vi "ABR-Initialize Stimulus.vi"(0 "Data folder":path, 5 "Npts":i32, 7 "Stimulus":T1={"Destination"="", "Waveform"=enum."TONE PIP", "Frequency (kHz)"=16.0, "Rep rate (/sec)"=30.0, "Alternate Polarity"=FALSE, "Sampling rate (Hz)"=100000.0, "Duration (ms)"=5.0, "Ramp (ms)"=0.5, "Click width (us)"=0.0, "ITI"=enum."Rate"} {"Frequency (kHz)" format="%.2f"}, 11 "error in (no error)":errorcluster) -> (4 "SigMan out":refnum<class "SignalManager.lvclass">, 15 "error out":errorcluster)   [LabVIEW 2020]
uses:
  epl-vi-lib/Signal Synthesis VIs/4th Generation/Classes/SignalManager/SignalManager.lvclass
  Typedefs/ABR-Stimulus.ctl
  epl-vi-lib/Signal Synthesis VIs/4th Generation/Classes/Channel/Channel.lvclass/Channel.ctl
  epl-vi-lib/Signal Synthesis VIs/4th Generation/Classes/Channel/Write Waveform.vi
  epl-vi-lib/Signal Synthesis VIs/4th Generation/Classes/Channel/Write Gate.vi
  epl-vi-lib/Signal Synthesis VIs/4th Generation/Classes/Channel/Write Level.vi
  epl-vi-lib/Signal Synthesis VIs/4th Generation/Classes/Channel/Write AltPol.vi
  epl-vi-lib/Signal Synthesis VIs/4th Generation/Classes/Waveforms/Tone/Tone.lvclass
  D:/Development/epl-vi-lib/Signal Synthesis VIs/4th Generation/Classes/Waveforms/Waveform/Waveform.lvclass
  epl-vi-lib/Signal Synthesis VIs/4th Generation/Classes/Waveforms/Pulse Train/Pulse Train.lvclass
  epl-vi-lib/Signal Synthesis VIs/4th Generation/Classes/Channel/Channel.lvclass
  epl-vi-lib/Signal Synthesis VIs/4th Generation/Classes/Level/Level.lvclass
  epl-vi-lib/Signal Synthesis VIs/4th Generation/Classes/Gate/Gate.lvclass
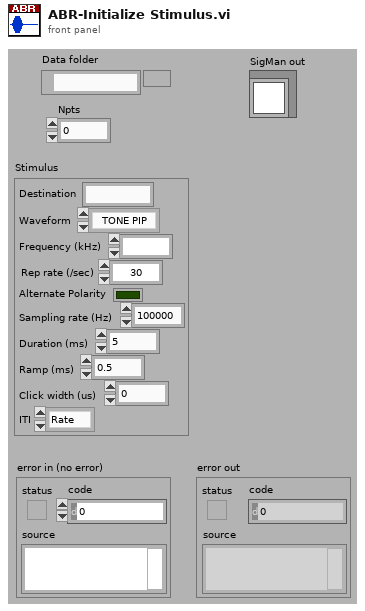
[diagram p1: front panel]
types:
  T1 = typedef "ABR-Stimulus.ctl" = cluster{"Destination":string, "Waveform":enum16{"TONE PIP", "CLICK"}, "Frequency (kHz)":ext, "Rep rate (/sec)":dbl, "Alternate Polarity":bool, "Sampling rate (Hz)":dbl, "Duration (ms)":dbl, "Ramp (ms)":dbl, "Click width (us)":dbl, "ITI":enum16{"Rate", "Interval"}}
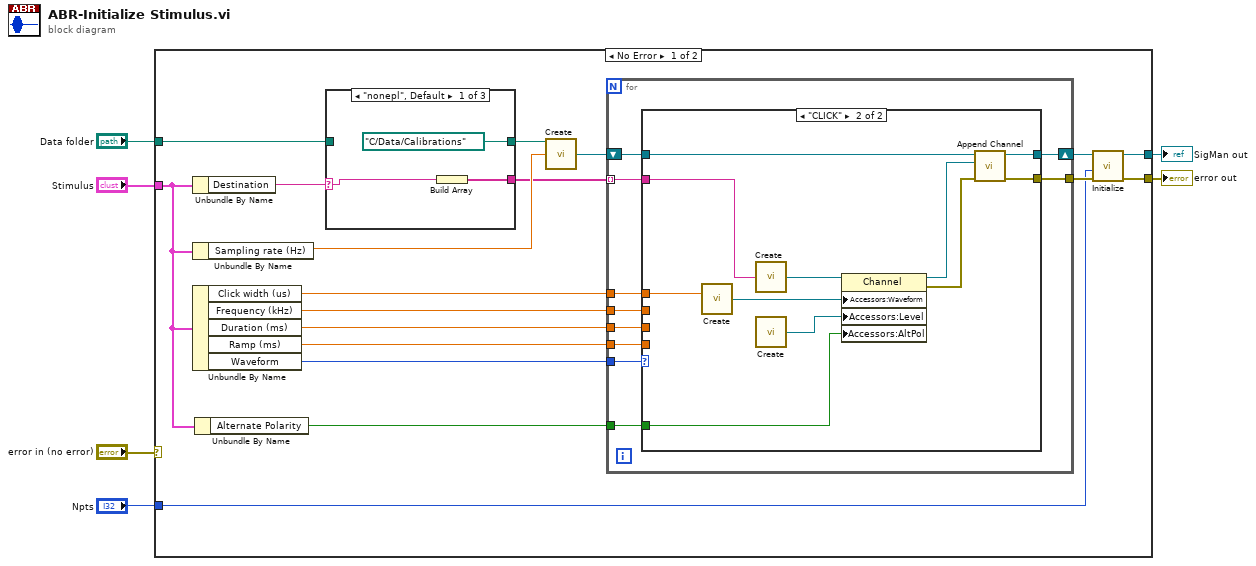
[diagram p0: block diagram]
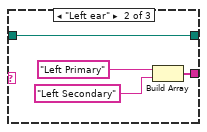
[diagram p2: hidden frame]
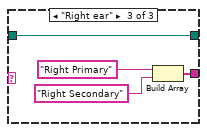
[diagram p3: hidden frame]
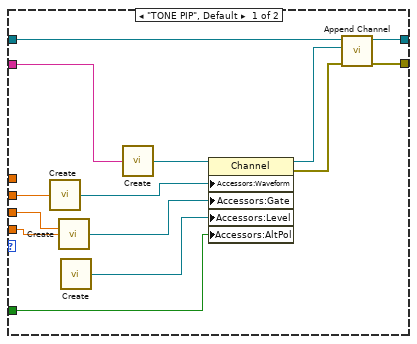
[diagram p4: hidden frame]
diagram:
  n1 = case shown="No Error" "error in (no error)" {
    selector: "error in (no error)" -> [_ w71]
    tunnel: [w12 w71] -> w6
    tunnel: "Stimulus" -> [w8 _]
    tunnel: "Data folder" -> [w19 _]
    tunnel: [w10 _] -> w2
    tunnel: "Npts" -> [w9 _]
    frame No Error {
      n2 = Unbundle By Name(w8) -> ("Destination"=w20:string)
      n3 = Unbundle By Name(w8) -> ("Sampling rate (Hz)"=w17:dbl)
      n4 = Unbundle By Name(w8) -> ("Click width (us)"=w11:dbl, "Frequency (kHz)"=w22:ext, "Duration (ms)"=w24:dbl, "Ramp (ms)"=w23:dbl, "Waveform"=w21:enum16{"TONE PIP", "CLICK"})
      n5 = Unbundle By Name(w8) -> ("Alternate Polarity"=w7:bool)
      n6 = case shown="\"nonepl\", Default" w20 {
        selector: w20 -> [w26 _ _]
        tunnel: [w25 w29 w33] -> w15
        tunnel: [path "C:/Data/Calibrations" ("Data folder") w28 w32] -> w18
        tunnel: w19 -> [_ w28 w32]
        frame "nonepl", Default {
          n7 = Build Array(w26) -> (w25:string[])
        }
        frame "Left ear" {
          n8 = Build Array("Left Primary", "Left Secondary") -> (w29:string[])
        }
        frame "Right ear" {
          n9 = Build Array("Right Primary", "Right Secondary") -> (w33:string[])
        }
      }
      n10 = call "Create.vi"("Cal Folder"=w18, "Fs (Hz)"=w17) -> ("SigMan"=w16:refnum<class "SignalManager.lvclass">)  [unwired: 13 in]
      n11 = for {
        tunnel: w24 -> [w45]
        tunnel: w23 -> [w44]
        tunnel: w22 -> [w43]
        tunnel: w21 -> [w42]
        shift-right: [w40] -> w14
        shift-left: w16 -> [w41]
        tunnel: w15 -> [w39] mode=indexing
        tunnel: [w38] -> w13
        tunnel: w11 -> [w37]
        tunnel: w7 -> [w36]
        n12 = case shown="\"CLICK\"" w42 {
          tunnel: w45 -> [w56 _]
          tunnel: w44 -> [w55 _]
          tunnel: w43 -> [w54 _]
          tunnel: w41 -> [w51 w67]
          tunnel: [w49 w65] -> w40
          tunnel: w39 -> [w50 w66]
          tunnel: [w47 w63] -> w38
          tunnel: w37 -> [_ w61]
          tunnel: w36 -> [w46 w60]
          frame "TONE PIP", Default {
            n13 = call "Create.vi"("Frequency (kHz)"=w54) -> ("Tone"=w57:refnum<class "Tone.lvclass">)  [unwired: 14 in]
            n14 = call "Create.vi"("Duration (ms)"=w56, "Ramp (ms)"=w55) -> ("Gate"=w53:refnum<class "Gate.lvclass">)  [unwired: 13 in]
            n15 = call "Create.vi"() -> ("Level"=w52:refnum<class "Level.lvclass">)  [unwired: 15 in]
            n16 = call "Create.vi"("Name"=w50) -> ("Channel"=w59:refnum<class "Channel.lvclass">)  [unwired: 14 in]
            n17 = property class="Channel"(reference=w59, "Accessors:Waveform"=w57, "Accessors:Gate"=w53, "Accessors:Level"=w52, "Accessors:AltPol"=w46) -> (reference out=w58:refnum<class "Channel.lvclass">, error out=w48:errorcluster)  [unwired: 1 in]
            n18 = call "Append Channel.vi"("error in (no error)"=w48, "Channel"=w58, "SignalManager in"=w51) -> ("error out"=w47:errorcluster, "SignalManager out"=w49:refnum<class "SignalManager.lvclass">)  [unwired: 7 in]
          }
          frame "CLICK" {
            n19 = call "Create.vi"("Width (us)"=w61) -> ("Pulse Train"=w62:refnum<class "Pulse Train.lvclass">)  [unwired: 14 in]
            n20 = call "Create.vi"("Name"=w66) -> ("Channel"=w70:refnum<class "Channel.lvclass">)  [unwired: 14 in]
            n21 = call "Create.vi"() -> ("Level"=w68:refnum<class "Level.lvclass">)  [unwired: 15 in]
            n22 = property class="Channel"(reference=w70, "Accessors:Waveform"=w62, "Accessors:Level"=w68, "Accessors:AltPol"=w60) -> (reference out=w69:refnum<class "Channel.lvclass">, error out=w64:errorcluster)  [unwired: 1 in]
            n23 = call "Append Channel.vi"("error in (no error)"=w64, "Channel"=w69, "SignalManager in"=w67) -> ("error out"=w63:errorcluster, "SignalManager out"=w65:refnum<class "SignalManager.lvclass">)  [unwired: 7 in]
          }
        }
      }
      n24 = call "Initialize.vi"("error in (no error)"=w13, "Npts"=w9, "SigMan in"=w14) -> ("error out"=w12:errorcluster, "SigMan out"=w10:refnum<class "SignalManager.lvclass">)  [unwired: 7 in]
    }
    frame Error {
    }
  }
  "error out" <- w6
  "SigMan out" <- w2
